vi "打开文件.vi"(9 "测试人员":string, 11 "错误输入（无错误）":errorcluster) -> (1 "tdms文件输出":refnum<k34>, 3 "错误输出":errorcluster)   [LabVIEW 2021]
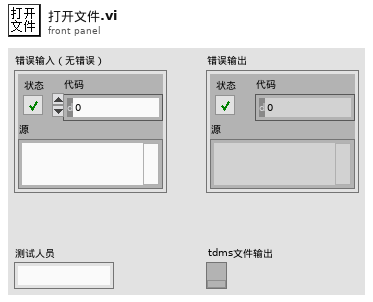
[diagram p1: front panel]
types:
  T1 = enum16{"open", "open or create", "create or replace", "create", "open (read-only)"}
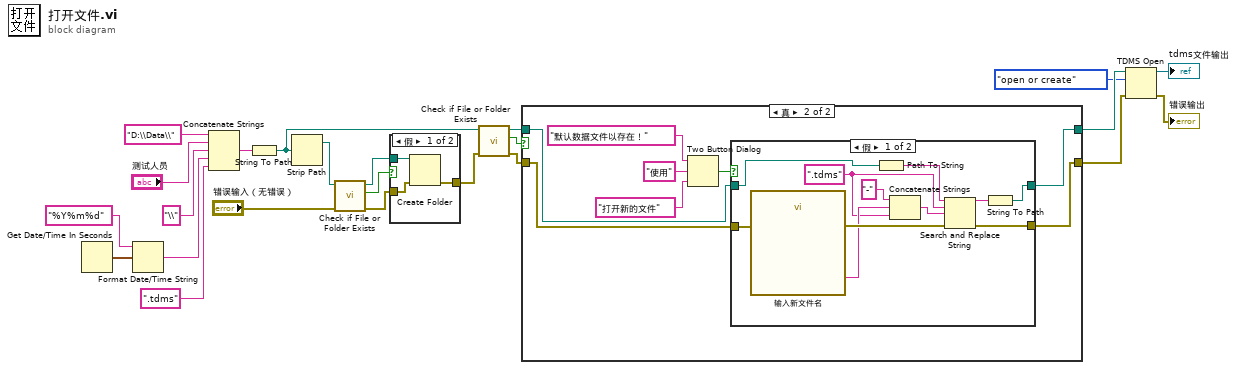
[diagram p0: block diagram]
diagram:
  n1 = Get Date/Time In Seconds() -> (seconds since 1Jan1904=w11:timestamp)
  n2 = Format Date/Time String(time format string (%c)="%Y%m%d" ("时间格式字符串(%c)"), seconds (now)=w11) -> (date/time string=w9:string)  [unwired: 1 in]
  n3 = Concatenate Strings("D:\\Data\\", "测试人员", "\\" ("字符串"), w9, ".tdms" ("字符串")) -> (w7:string)
  n4 = String To Path(string=w7) -> (path=w6:path)
  n5 = Strip Path(path=w6) -> (stripped path=w20:path)  [unwired: 1 out]
  n6 = call <vilib>:"Check if File or Folder Exists.vi"("error in (no error)"="错误输入（无错误）", "path"=w20) -> ("error out"=w18:errorcluster, "file or folder exists?"=w17:bool, "dup path"=w19:path)  [unwired: 7 in]
  n7 = case shown="假" w17 {
    tunnel: w19 -> [w26 _]
    tunnel: w18 -> [w25 w27]
    tunnel: [w24 w27] -> w16
    frame False {
      n8 = Create Folder(path (use dialog)=w26, error in=w25) -> (error out=w24:errorcluster)  [unwired: 1 in, 2 out]
    }
    frame True {
    }
  }
  n9 = call <vilib>:"Check if File or Folder Exists.vi"("error in (no error)"=w16, "path"=w6) -> ("error out"=w23:errorcluster, "file or folder exists?"=w22:bool, "dup path"=w21:path)  [unwired: 7 in]
  n10 = case shown="真" w22 {
    tunnel: w23 -> [w29 w33]
    tunnel: w21 -> [w28 w32]
    tunnel: [w29 w30] -> w4
    tunnel: [w28 w31] -> w5
    frame False {
    }
    frame True {
      n11 = Two Button Dialog(message="默认数据文件以存在！" ("消息"), 1:"打开新的文件" ("F按钮名称（“取消”）"), 2:"使用" ("T按钮名称（“确定”）")) -> (T button?=w34:bool)
      n12 = case shown="假" w34 {
        tunnel: w33 -> [w42 w49]
        tunnel: w32 -> [w41 w50]
        tunnel: [w39 w50] -> w31
        tunnel: [w38 w49] -> w30
        frame False {
          w43 = ".tdms" ("搜索字符串")
          n13 = call "输入新文件名"("error in (no error)"=w42) -> ("输入"=w45:string, "error out"=w47:errorcluster)  [unwired: 16 in, 1 out]
          n14 = Path To String(path=w41) -> (string=w40:string)
          n15 = Concatenate Strings("-" ("字符串"), w45, w43) -> (w46:string)
          n16 = Search and Replace String(input string=w40, search string=w43, replace string=w46, error in=w47) -> (result string=w48:string, error out=w38:errorcluster)  [unwired: 4 in, 2 out]
          n17 = String To Path(string=w48) -> (path=w39:path)
        }
        frame True {
        }
      }
    }
  }
  n18 = TDMS Open(8:w4, 10:T1."open or create" ("操作(0:open)"), 11:w5) -> (0:→"错误输出":errorcluster, 3:→"tdms文件输出":refnum<k34>)  [unwired: 4 in]
